vi "StringToCoord.vi"(1 "String coordinates":string) -> (0 "coordinates":dbl[](array[numeric]) format="%.2f")   [LabVIEW 2013, in "File management.lvlib"]
uses:
  File management.lvlib
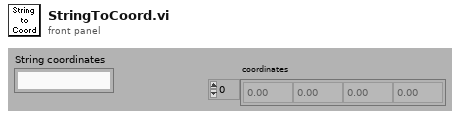
[diagram p1: front panel]
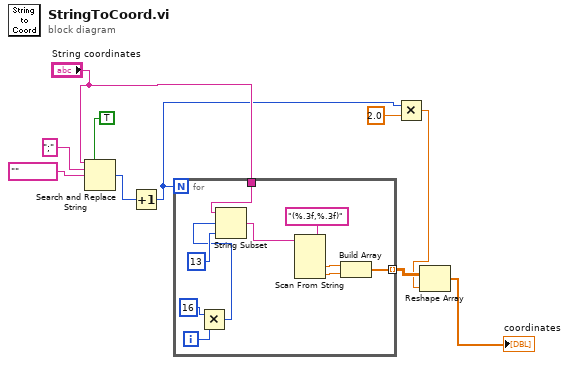
[diagram p0: block diagram]
diagram:
  n1 = Search and Replace String(replace all?=TRUE ("tout remplacer ? (F)"), input string="String coordinates", search string=";" ("chaîne recherchée"), replace string="" ("chaîne de remplacement (\"\")")) -> (number of replacements=w3:i32)  [unwired: 1 in, 6 out]
  n2 = Increment(x=w3) -> (x+1=w2:i32)
  n3 = for {
    N: w2 -> [_]
    tunnel: "String coordinates" -> [w20]
    tunnel: [w11] -> w10 mode=indexing
    i -> [w18]
    n4 = Multiply(x=16, y=w18) -> (x*y=w16:i32)
    n5 = String Subset(string=w20, offset (0)=w16, length (rest)=13 ("length (rest)")) -> (substring=w12:string)
    n6 = Scan From String(format string="(%.3f,%.3f)", input string=w12) -> (output 1=w14:dbl, output 2=w15:dbl)  [unwired: 2 in, 5 out]
    n7 = Build Array(w14, w15) -> (w11:dbl[])
  }
  n8 = Multiply(x=w2, y=2.0) -> (x*y=w8:dbl)
  n9 = Reshape Array(w10, w8) -> (→"coordinates":dbl[])
